vi "CTRE_CANifier_GetQuadratureSensor.vi"(8 "error in":errorcluster, 11 "CANifierDevRef":T1) -> (0 "error out":errorcluster, 1 "vel":i32, 2 "pos":i32, 3 "CANifierDevRef":T1)   [LabVIEW 2019]
uses:
  <vilib>/Rock Robotics/WPI/ThirdParty/Phoenix-LabVIEW/CANifier/CTRE_CANifier_DeviceRef.ctl
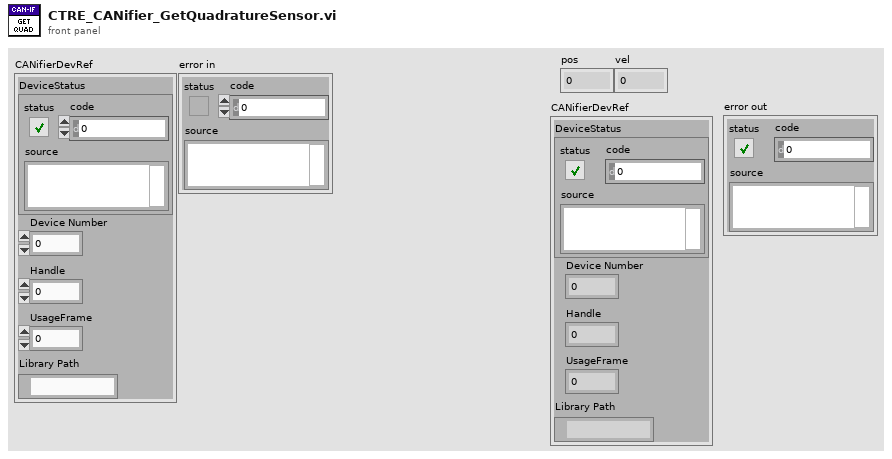
[diagram p1: front panel]
types:
  T1 = typedef "CTRE_CANifier_DeviceRef.ctl" = cluster{"DeviceStatus":errorcluster, "Device Number":u8, "Handle":u64, "UsageFrame":u32, "Library Path":path}
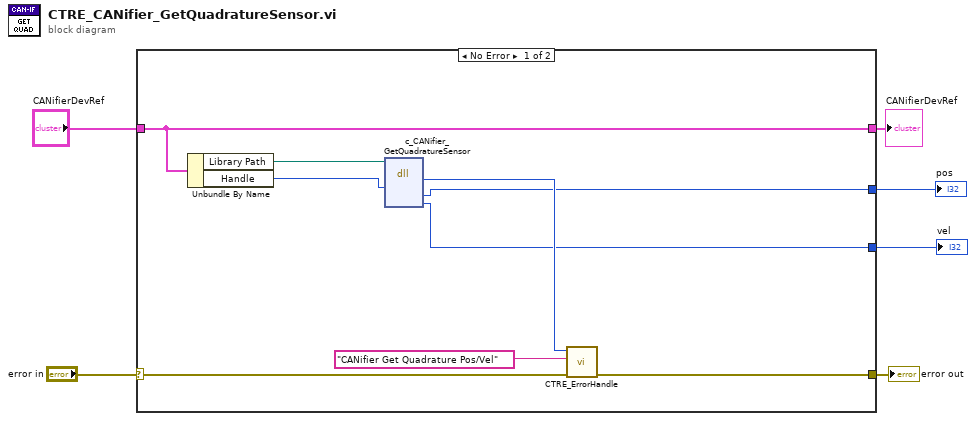
[diagram p0: block diagram]
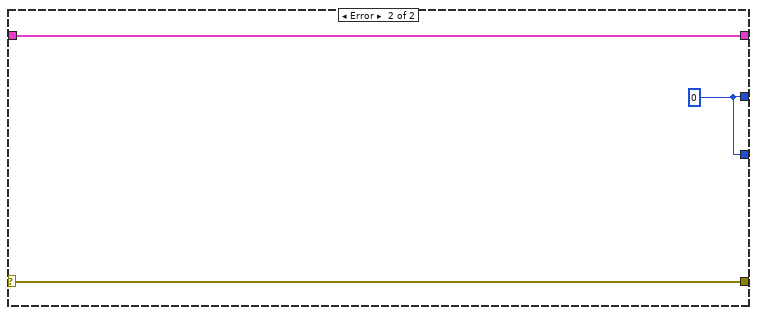
[diagram p2: hidden frame]
diagram:
  n1 = case shown="No Error" "error in" {
    selector: "error in" -> [w10 w17]
    tunnel: "CANifierDevRef" -> [w13 w18]
    tunnel: [w13 w18] -> w4
    tunnel: [w11 w17] -> w3
    tunnel: [w8 w16] -> w2
    tunnel: [w7 w16] -> w1
    frame No Error {
      n2 = Unbundle By Name(w13) -> ("Library Path"=w15:path, "Handle"=w14:u64)
      n3 = dll-call lib="?" fn="c_CANifier_GetQuadratureSensor"(path in=w15, "handle"=w14) -> ("CTR_Code"=w12:i8, "pos"=w7:i32, "vel"=w8:i32)  [unwired: 5 in, 2 out]
      n4 = call <vilib>:"CTRE_ErrorHandle.vi"("error in"=w10, "origin"="CANifier Get Quadrature Pos/Vel", "code"=w12) -> ("error out"=w11:errorcluster)  [unwired: 8 in]
    }
    frame Error {
      w16 = 0 ("pos")
    }
  }
  "CANifierDevRef" <- w4
  "error out" <- w3
  "pos" <- w1
  "vel" <- w2
